vi "AO_Volt_and_Curr.vi"(6 "Curnt_Value":dbl[](array[numeric]) format="%0.2f", 7 "Volt_Value":dbl[](array[numeric]) format="%0.2f", 9 "Current Channel":string[](array[string]), 10 "Volt Channel":string[](array[string])) -> (0 "error out":errorcluster)   [LabVIEW 2017]
uses:
  <vilib>/DAQmx/write.llb/DAQmx Write (Analog 1D DBL NChan 1Samp).vi
  <vilib>/DAQmx/create/channels.llb/DAQmx Create Channel (AO-Voltage-Basic).vi
  <vilib>/DAQmx/miscellaneous.llb/DAQmx Fill In Error Info.vi
  <vilib>/DAQmx/create/channels.llb/DAQmx Create Channel (AO-Current-Basic).vi
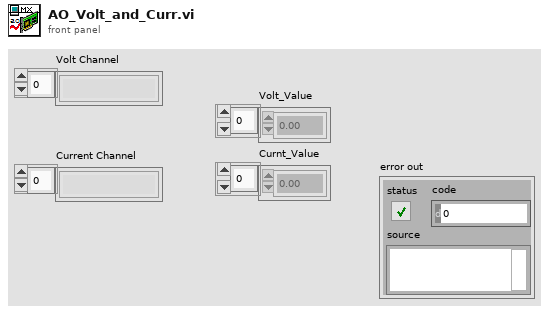
[diagram p1: front panel]
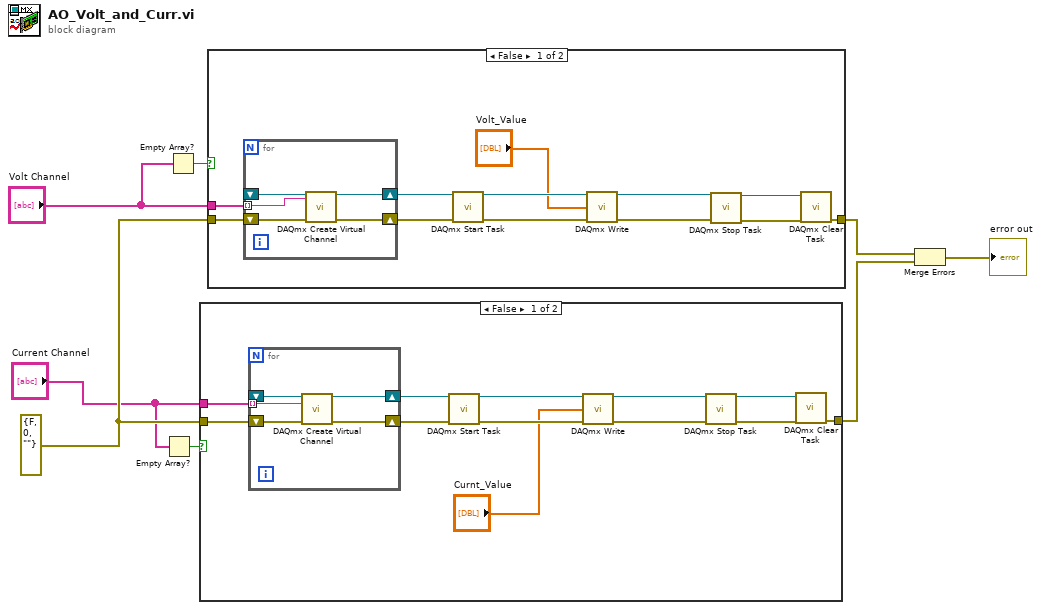
[diagram p0: block diagram]
diagram:
  w6 = errorcluster {"status"=FALSE, "code"=0, "source"=""} ("error out")
  n1 = Empty Array?(array="Current Channel") -> (empty?=w4:bool)
  n2 = Empty Array?(array="Volt Channel") -> (empty?=w2:bool)
  n3 = case shown="False" w4 {
    tunnel: [w12 w26] -> w7
    tunnel: w6 -> [w10 w26]
    tunnel: "Current Channel" -> [w9 _]
    frame False {
      n4 = for {
        shift-right: [w25] -> w18
        shift-left: _ -> [w23]
        shift-right: [w24] -> w17
        shift-left: w10 -> [w22]
        tunnel: w9 -> [w21] mode=indexing
        n5 = call-poly <vilib>:"DAQmx Create Virtual Channel.vi"("task in"=w23, "physical channels"=w21, "error in"=w22) -> ("task out"=w25:refnum<k21>, "error out"=w24:errorcluster)  [unwired: 11 in]
      }
      n6 = call <vilib>:"DAQmx Start Task.vi"("task/channels in"=w18, "error in"=w17) -> ("task out"=w19:refnum<k21>, "error out"=w20:errorcluster)  [unwired: 12 in]
      n7 = call-poly <vilib>:"DAQmx Write.vi"("task/channels in"=w19, "data"="Curnt_Value", "error in"=w20) -> ("task out"=w14:refnum<k21>, "error out"=w13:errorcluster)  [unwired: 10 in, 1 out]
      n8 = call <vilib>:"DAQmx Stop Task.vi"("task/channels in"=w14, "error in"=w13) -> ("task out"=w16:refnum<k21>, "error out"=w15:errorcluster)  [unwired: 12 in]
      n9 = call <vilib>:"DAQmx Clear Task.vi"("task in"=w16, "error in"=w15) -> ("error out"=w12:errorcluster)  [unwired: 13 in]
    }
    frame True {
      # "没有选择电流输出通道！"
    }
  }
  n10 = case shown="False" w2 {
    tunnel: [w30 w44] -> w8
    tunnel: w6 -> [w28 w44]
    tunnel: "Volt Channel" -> [w27 _]
    frame False {
      n11 = for {
        shift-right: [w43] -> w38
        shift-left: _ -> [w41]
        shift-right: [w42] -> w37
        shift-left: w28 -> [w40]
        tunnel: w27 -> [w39] mode=indexing
        n12 = call-poly <vilib>:"DAQmx Create Virtual Channel.vi"("task in"=w41, "physical channels"=w39, "error in"=w40) -> ("task out"=w43:refnum<k21>, "error out"=w42:errorcluster)  [unwired: 11 in]
      }
      n13 = call <vilib>:"DAQmx Start Task.vi"("task/channels in"=w38, "error in"=w37) -> ("task out"=w36:refnum<k21>, "error out"=w35:errorcluster)  [unwired: 12 in]
      n14 = call-poly <vilib>:"DAQmx Write.vi"("task/channels in"=w36, "data"="Volt_Value", "error in"=w35) -> ("task out"=w34:refnum<k21>, "error out"=w33:errorcluster)  [unwired: 10 in, 1 out]
      n15 = call <vilib>:"DAQmx Stop Task.vi"("task/channels in"=w34, "error in"=w33) -> ("task out"=w31:refnum<k21>, "error out"=w32:errorcluster)  [unwired: 12 in]
      n16 = call <vilib>:"DAQmx Clear Task.vi"("task in"=w31, "error in"=w32) -> ("error out"=w30:errorcluster)  [unwired: 13 in]
    }
    frame True {
      # "没有选择电压输出通道！"
    }
  }
  n17 = Merge Errors(w8, w7) -> (→"error out":errorcluster)
